vi "FWCS_Stream.vi"() -> ()   [LabVIEW 2018]
uses:
  Stream/Stream.lvclass
  RxTx/RxTx.lvclass
  Stream/Stream.lvclass/Stream.ctl
panel:
  out "error out 2":errorcluster
  out "error out":errorcluster
  in  "RxTx.lvclass":refnum<class "RxTx.lvclass">
  in  "Stream.lvclass":refnum<class "Stream.lvclass">
  in  "RxTx.lvclass 2":refnum<class "RxTx.lvclass">
  in  "Stream.lvclass 2":refnum<class "Stream.lvclass">
  # "Filter Wheel Stream Communication"
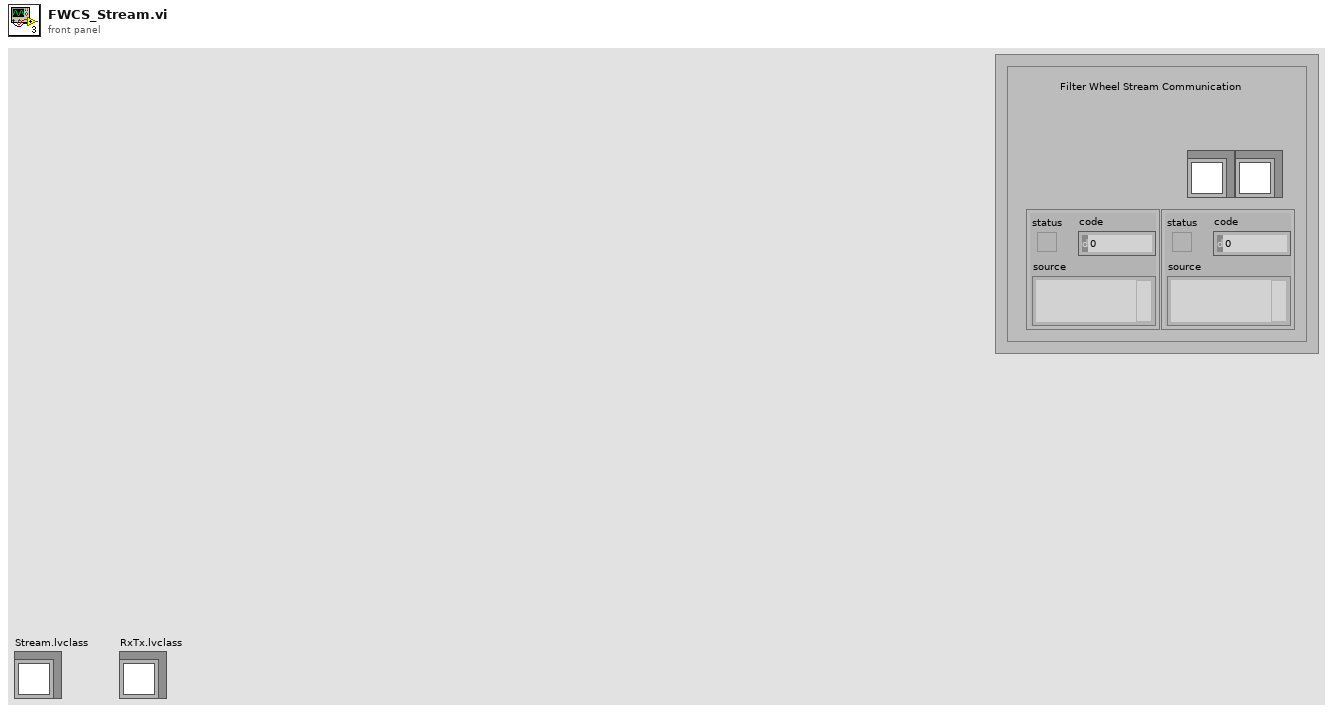
[diagram p1: front panel]
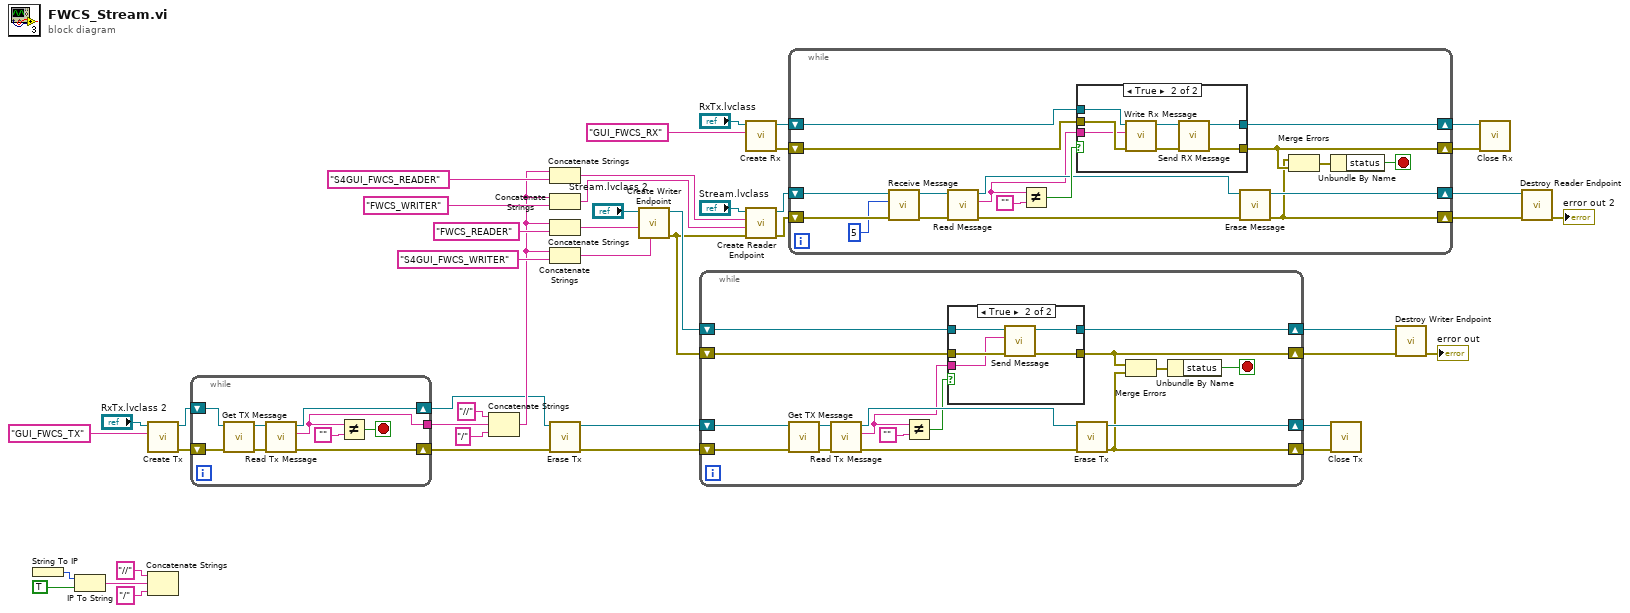
[diagram p0: block diagram]
diagram:
  n1 = String To IP() -> (0:w21:u32)  [unwired: 1 in]
  n2 = IP To String(1:TRUE ("dot notation? (F)"), 2:w21) -> (0:w18:string)
  n3 = call "Create Tx.vi"("Writer Name"="GUI_FWCS_TX" ("Reader Name"), "RxTx in"="RxTx.lvclass 2") -> ("error out"=w2:errorcluster, "RxTx out"=w3:refnum<class "RxTx.lvclass">)  [unwired: 8 in]
  n4 = Concatenate Strings("//" ("Reader Name"), w18, "/" ("Reader Name")) -> ()  [unwired: 1 out]
  n5 = while {
    shift-right: [w51] -> w7
    shift-left: w2 -> [w48]
    shift-right: [w52] -> w6
    shift-left: w3 -> [w47]
    tunnel: [w46] -> w1
    stop <- w53 stop-if-true
    n6 = call "Get TX Message.vi"("error in (no error)"=w48, "RxTx in"=w47) -> ("error out"=w49:errorcluster, "RxTx out"=w50:refnum<class "RxTx.lvclass">)  [unwired: 8 in]
    n7 = call "Read Tx Message.vi"("error in (no error)"=w49, "RxTx in"=w50) -> ("error out"=w51:errorcluster, "Tx Message"=w46:string, "RxTx out"=w52:refnum<class "RxTx.lvclass">)  [unwired: 7 in]
    n8 = Not Equal?(x=w46, y="") -> (x != y?=w53:bool)
  }
  n9 = Concatenate Strings("//" ("Reader Name"), w1, "/" ("Reader Name")) -> (w8:string)
  n10 = Concatenate Strings(w8, "S4GUI_FWCS_READER" ("Reader Name")) -> (w27:string)
  n11 = Concatenate Strings(w8, "FWCS_WRITER" ("reader name")) -> (w13:string)
  n12 = Concatenate Strings(w8, "FWCS_READER" ("Reader Name")) -> (w12:string)
  n13 = Concatenate Strings(w8, "S4GUI_FWCS_WRITER" ("reader name")) -> (w36:string)
  n14 = call "Erase Tx.vi"("error in (no error)"=w7, "RxTx in"=w6) -> ("error out"=w4:errorcluster, "RxTx out"=w5:refnum<class "RxTx.lvclass">)  [unwired: 8 in]
  n15 = call "Create Writer Endpoint.vi"("writer name"=w36, "reader name"=w12, "Stream in"="Stream.lvclass 2") -> ("error out"=w22:errorcluster, "Stream out"=w42:refnum<class "Stream.lvclass">)  [unwired: 7 in]
  n16 = while {
    shift-right: [w64] -> w40
    shift-left: w22 -> [w66]
    shift-right: [w65] -> w45
    shift-left: w42 -> [w67]
    shift-right: [w59] -> w43
    shift-left: w4 -> [w68]
    shift-right: [w61] -> w44
    shift-left: w5 -> [w69]
    stop <- w56 stop-if-true
    n17 = call "Get TX Message.vi"("error in (no error)"=w68, "RxTx in"=w69) -> ("error out"=w70:errorcluster, "RxTx out"=w57:refnum<class "RxTx.lvclass">)  [unwired: 8 in]
    n18 = call "Read Tx Message.vi"("error in (no error)"=w70, "RxTx in"=w57) -> ("error out"=w60:errorcluster, "Tx Message"=w55:string, "RxTx out"=w62:refnum<class "RxTx.lvclass">)  [unwired: 7 in]
    n19 = Not Equal?(x=w55, y="") -> (x != y?=w58:bool)
    n20 = case shown="True" w58 {
      tunnel: w67 -> [w73 w78]
      tunnel: w66 -> [w72 w77]
      tunnel: [w73 w76] -> w65
      tunnel: w55 -> [_ w75]
      tunnel: [w72 w74] -> w64
      frame False {
      }
      frame True {
        n21 = call "Send Message.vi"("error in (no error)"=w77, "Message"=w75, "Stream in"=w78) -> ("error out"=w74:errorcluster, "Stream out"=w76:refnum<class "Stream.lvclass">)  [unwired: 7 in]
      }
    }
    n22 = call "Erase Tx.vi"("error in (no error)"=w60, "RxTx in"=w62) -> ("error out"=w59:errorcluster, "RxTx out"=w61:refnum<class "RxTx.lvclass">)  [unwired: 8 in]
    n23 = Merge Errors(w64, w59) -> (w71:errorcluster)
    n24 = Unbundle By Name(w71) -> ("status"=w56:bool)
  }
  n25 = call "Create Rx.vi"("Reader Name"="GUI_FWCS_RX", "RxTx in"="RxTx.lvclass") -> ("error out"=w24:errorcluster, "RxTx out"=w25:refnum<class "RxTx.lvclass">)  [unwired: 8 in]
  n26 = call "Create Reader Endpoint.vi"("error in (no error)"=w22, "writer name"=w13, "reader name"=w27, "Stream in"="Stream.lvclass") -> ("error out"=w30:errorcluster, "Stream out"=w32:refnum<class "Stream.lvclass">)  [unwired: 6 in]
  n27 = while {
    shift-right: [w79] -> w29
    shift-left: w30 -> [w93]
    shift-right: [w82] -> w35
    shift-left: w32 -> [w94]
    shift-right: [w84] -> w33
    shift-left: w24 -> [w86]
    shift-right: [w85] -> w34
    shift-left: w25 -> [w87]
    stop <- w95 stop-if-true
    n28 = call "Receive Message.vi"("error in (no error)"=w93, "timeout ms"=5, "Stream in"=w94) -> ("error out"=w91:errorcluster, "Stream out"=w90:refnum<class "Stream.lvclass">)  [unwired: 7 in]
    n29 = call "Read Message.vi"("error in (no error)"=w91, "Stream in"=w90) -> ("error out"=w83:errorcluster, "Message"=w80:string, "Stream out"=w81:refnum<class "Stream.lvclass">)  [unwired: 7 in]
    n30 = Not Equal?(x=w80, y="") -> (x != y?=w89:bool)
    n31 = case shown="True" w89 {
      tunnel: w87 -> [w98 w105]
      tunnel: w86 -> [w97 w104]
      tunnel: [w98 w101] -> w85
      tunnel: [w97 w100] -> w84
      tunnel: w80 -> [_ w99]
      frame False {
      }
      frame True {
        n32 = call "Write Rx Message.vi"("error in (no error)"=w104, "Rx Message"=w99, "RxTx in"=w105) -> ("error out"=w103:errorcluster, "RxTx out"=w102:refnum<class "RxTx.lvclass">)  [unwired: 7 in]
        n33 = call "Send RX Message.vi"("error in (no error)"=w103, "RxTx in"=w102) -> ("error out"=w100:errorcluster, "RxTx out"=w101:refnum<class "RxTx.lvclass">)  [unwired: 8 in]
      }
    }
    n34 = call "Erase Message.vi"("error in (no error)"=w83, "Stream in"=w81) -> ("error out"=w79:errorcluster, "Stream out"=w82:refnum<class "Stream.lvclass">)  [unwired: 8 in]
    n35 = Merge Errors(w79, w84) -> (w96:errorcluster)
    n36 = Unbundle By Name(w96) -> ("status"=w95:bool)
  }
  n37 = call "Close Tx.vi"("error in (no error)"=w43, "RxTx in"=w44) -> ()  [unwired: 8 in, 2 out]
  n38 = call "Destroy Writer Endpoint.vi"("error in (no error)"=w40, "Stream in"=w45) -> ("error out"=→"error out":errorcluster)  [unwired: 8 in, 1 out]
  n39 = call "Close Rx.vi"("error in (no error)"=w33, "RxTx in"=w34) -> ()  [unwired: 8 in, 2 out]
  n40 = call "Destroy Reader Endpoint.vi"("error in (no error)"=w29, "Stream in"=w35) -> ("error out"=→"error out 2":errorcluster)  [unwired: 8 in, 1 out]
